vi "_test Engine Lock.vi"() -> ()   [LabVIEW 2012]
uses:
  Engine/Move Speed.ctl
panel:
  in  "Move Speed (Normal)":T1
  out "GObject":bool
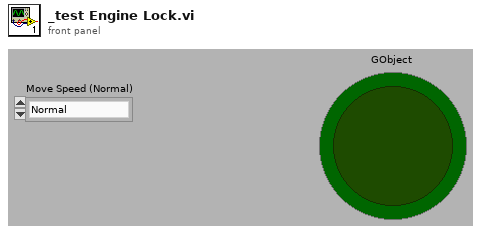
[diagram p1: front panel]
types:
  T1 = typedef "Move Speed.ctl" = enum16{"Normal", "Fast", "Slow", "Instantaneous"}
  T2 = typedef "LVPoint32TypeDef.ctl" = cluster{"Horizontal":i32, "Vertical":i32}
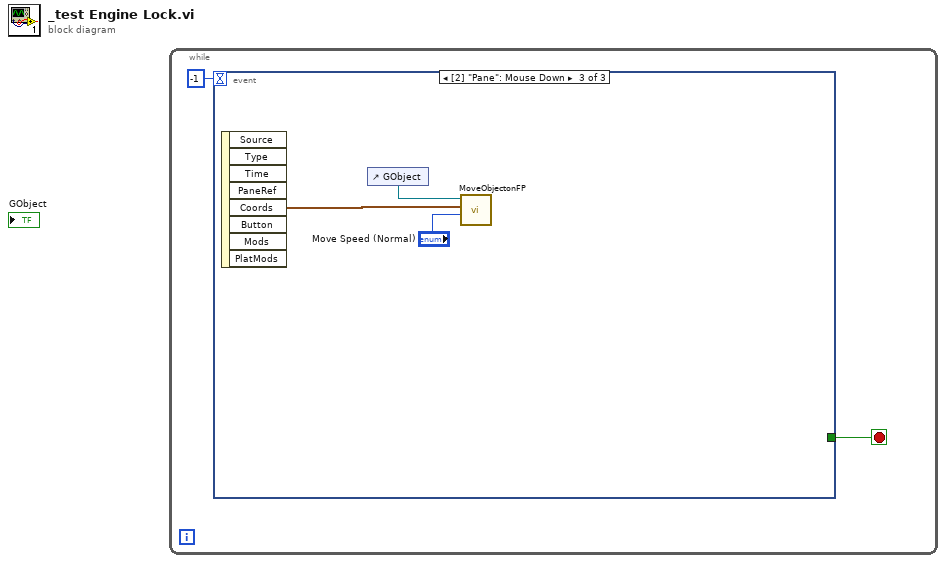
[diagram p0: block diagram]
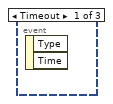
[diagram p2: hidden frame]
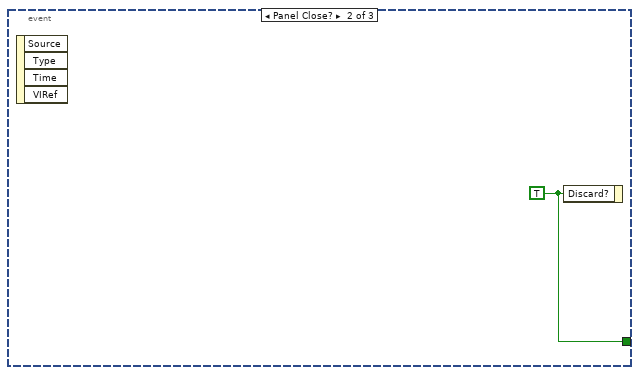
[diagram p3: hidden frame]
diagram:
  n1 = while {
    stop <- w1 stop-if-true
    n2 = event shown="[2] \"Pane\": Mouse Down" {
      selector: _ -> [_ _ _]
      dyn-events: _ -> [_ _ _]
      timeout: -1 -> [_ _ _]
      tunnel: [_ w3 _] -> w1
      event Timeout {
        n3 = event-data() -> ()  [unwired: 3 out]
      }
      event Panel Close? {
        w3 = TRUE ("Discard?")
        n4 = event-data() -> ()  [unwired: 5 out]
        n5 = event-data("Discard?"=w3) -> ()  [unwired: 1 in, 1 out]
      }
      event Mouse Down {
        n6 = event-data() -> ("Coords"=w5:T2)  [unwired: 8 out]
        n7 = control-ref of="GObject"() -> (w6:refnum<vi>)
        n8 = call "MoveObjectonFP.vi"("Move Speed (Instantaneous)"="Move Speed (Normal)", "Center Position for Object"=w5, "GObject"=w6) -> ()  [unwired: 2 in, 7 out]
      }
    }
  }
